vi "DivU16toU8.vi"(0 "Uint16_in":u16 format="%x") -> (1 "Uint8L_out":u8 format="%x", 2 "Uint8H_out":u8 format="%x")   [LabVIEW 2015]
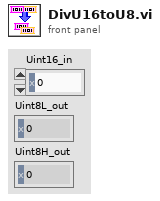
[diagram p1: front panel]
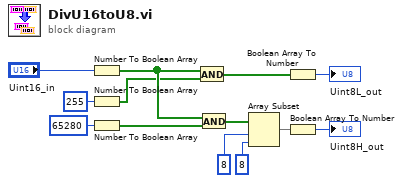
[diagram p0: block diagram]
diagram:
  n1 = Number To Boolean Array(number="Uint16_in") -> (Boolean array=w12:bool[])
  n2 = Number To Boolean Array(number=u16 255 ("BYTE 20")) -> (Boolean array=w9:bool[])
  n3 = Number To Boolean Array(number=u16 65280 ("BYTE 21")) -> (Boolean array=w8:bool[])
  n4 = And(x=w12, y=w9) -> (x .and. y?=w7:bool[])
  n5 = And(x=w12, y=w8) -> (x .and. y?=w1:bool[])
  n6 = Array Subset(array=w1, index=8, length=8) -> (w2:bool[])
  n7 = Boolean Array To Number(Boolean array=w7) -> (number=→"Uint8L_out":u32)
  n8 = Boolean Array To Number(Boolean array=w2) -> (number=→"Uint8H_out":u32)
